vi "lib Variant to String.vi"(8 "error in (no error)":errorcluster, 11 "Variant":variant) -> (0 "error out":errorcluster, 3 "String":string)   [LabVIEW 2018]
uses:
  <vilib>/Utility/Data Type/NI_Data Type.lvlib
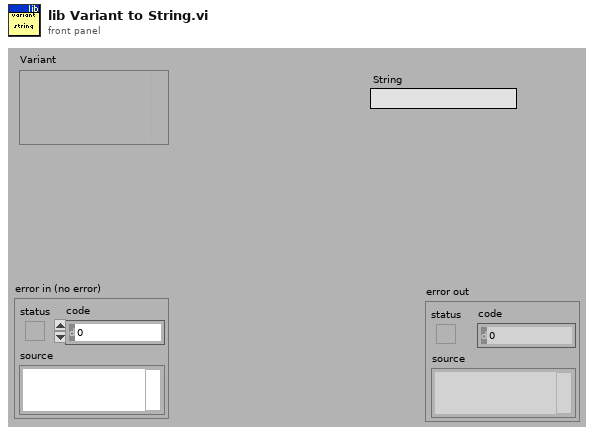
[diagram p1: front panel]
types:
  T1 = typedef "NI_Data Type.lvlib/Data Type.ctl" = enum8{"Invalid Type", "Void", "I8", "I16", "I32", "I64", "U8", "U16", "U32", "U64", "Single Float", "Double Float", "Extended Float", "Single Complex", "Double Complex", "Extended Complex", "Enum U8", "Enum U16", "Enum U32", "Enum U64", "Single Float With Unit", "Double Float With Unit", "Extended Float With Unit", "Single Complex with Unit", "Double Complex with Unit", "Extended Complex with Unit", "Boolean", "String", "Path", "Picture", "Tag", "Array", "Cluster", "Variant", "LV Variant", "Waveform", "Timestamp", "Digital Waveform", "Digital Data", "ExpressData", "Refnum", "External Data", "VI", "Poly VI", "LabVIEW Class Instance", "Fixed Point"}
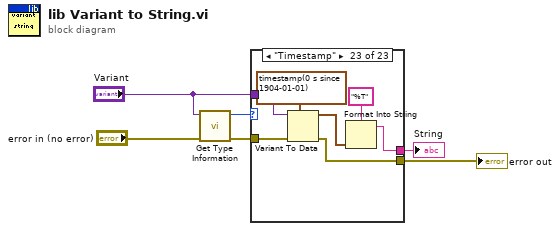
[diagram p0: block diagram]
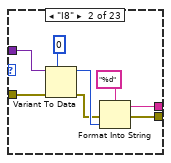
[diagram p3: hidden frame]
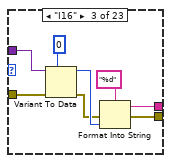
[diagram p4: hidden frame]
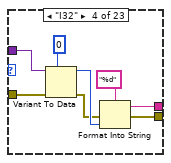
[diagram p5: hidden frame]
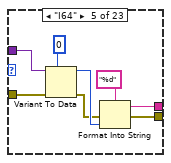
[diagram p6: hidden frame]
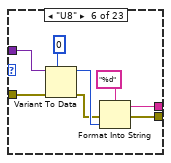
[diagram p7: hidden frame]
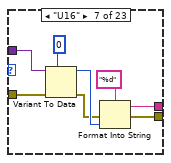
[diagram p8: hidden frame]
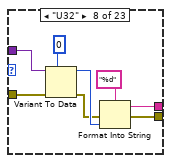
[diagram p9: hidden frame]
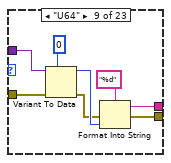
[diagram p10: hidden frame]
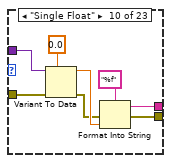
[diagram p11: hidden frame]
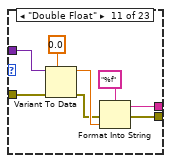
[diagram p12: hidden frame]
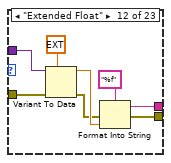
[diagram p13: hidden frame]
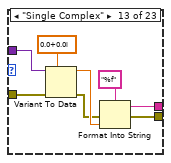
[diagram p14: hidden frame]
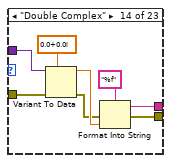
[diagram p15: hidden frame]
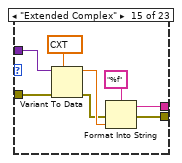
[diagram p16: hidden frame]
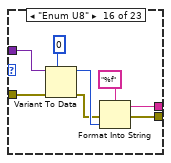
[diagram p17: hidden frame]
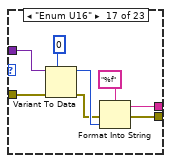
[diagram p18: hidden frame]
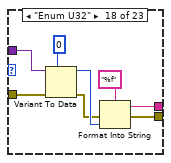
[diagram p19: hidden frame]
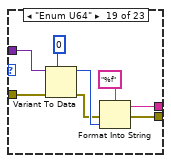
[diagram p20: hidden frame]
diagram:
  n1 = call <vilib>:"Get Type Information.vi"("error in (no error)"="error in (no error)", "Variant"="Variant") -> ("error out"=w5:errorcluster, "Type"=w6:T1)  [unwired: 5 in, 3 out]
  n2 = case shown="\"Timestamp\"" w6 {
    tunnel: "Variant" -> [_ w14 w22 w30 w38 w46 w54 w62 w70 w78 w86 w94 w102 w110 w118 w126 w134 w142 w150 w158 w163 w169 w176]
    tunnel: [_ w11 w19 w27 w35 w43 w51 w59 w67 w75 w83 w91 w99 w107 w115 w123 w131 w139 w147 w155 w160 w165 w171] -> w1
    tunnel: w5 -> [w7 w10 w18 w26 w34 w42 w50 w58 w66 w74 w82 w90 w98 w106 w114 w122 w130 w138 w146 w154 w162 w168 w175]
    tunnel: [w7 w8 w16 w24 w32 w40 w48 w56 w64 w72 w80 w88 w96 w104 w112 w120 w128 w136 w144 w152 w161 w166 w174] -> w2
    frame "Invalid Type", Default {
    }
    frame "I8" {
      n3 = Variant To Data(error in=w10, type=i8 0, Variant=w14) -> (data=w12:i8, error out=w9:errorcluster)
      n4 = Format Into String(format string="%d", error in=w9, w12) -> (resulting string=w11:string, error out=w8:errorcluster)  [unwired: 1 in]
    }
    frame "I16" {
      n5 = Variant To Data(error in=w18, type=i16 0, Variant=w22) -> (data=w20:i16, error out=w17:errorcluster)
      n6 = Format Into String(format string="%d", error in=w17, w20) -> (resulting string=w19:string, error out=w16:errorcluster)  [unwired: 1 in]
    }
    frame "I32" {
      n7 = Variant To Data(error in=w26, type=0, Variant=w30) -> (data=w28:i32, error out=w25:errorcluster)
      n8 = Format Into String(format string="%d", error in=w25, w28) -> (resulting string=w27:string, error out=w24:errorcluster)  [unwired: 1 in]
    }
    frame "I64" {
      n9 = Variant To Data(error in=w34, type=i64 0, Variant=w38) -> (data=w36:i64, error out=w33:errorcluster)
      n10 = Format Into String(format string="%d", error in=w33, w36) -> (resulting string=w35:string, error out=w32:errorcluster)  [unwired: 1 in]
    }
    frame "U8" {
      n11 = Variant To Data(error in=w42, type=u8 0, Variant=w46) -> (data=w44:u8, error out=w41:errorcluster)
      n12 = Format Into String(format string="%d", error in=w41, w44) -> (resulting string=w43:string, error out=w40:errorcluster)  [unwired: 1 in]
    }
    frame "U16" {
      n13 = Variant To Data(error in=w50, type=u16 0, Variant=w54) -> (data=w52:u16, error out=w49:errorcluster)
      n14 = Format Into String(format string="%d", error in=w49, w52) -> (resulting string=w51:string, error out=w48:errorcluster)  [unwired: 1 in]
    }
    frame "U32" {
      n15 = Variant To Data(error in=w58, type=u32 0, Variant=w62) -> (data=w60:u32, error out=w57:errorcluster)
      n16 = Format Into String(format string="%d", error in=w57, w60) -> (resulting string=w59:string, error out=w56:errorcluster)  [unwired: 1 in]
    }
    frame "U64" {
      n17 = Variant To Data(error in=w66, type=u64 0, Variant=w70) -> (data=w68:u64, error out=w65:errorcluster)
      n18 = Format Into String(format string="%d", error in=w65, w68) -> (resulting string=w67:string, error out=w64:errorcluster)  [unwired: 1 in]
    }
    frame "Single Float" {
      n19 = Variant To Data(error in=w74, type=sgl 0.0, Variant=w78) -> (data=w76:sgl, error out=w73:errorcluster)
      n20 = Format Into String(format string="%f", error in=w73, w76) -> (resulting string=w75:string, error out=w72:errorcluster)  [unwired: 1 in]
    }
    frame "Double Float" {
      n21 = Variant To Data(error in=w82, type=0.0, Variant=w86) -> (data=w84:dbl, error out=w81:errorcluster)
      n22 = Format Into String(format string="%f", error in=w81, w84) -> (resulting string=w83:string, error out=w80:errorcluster)  [unwired: 1 in]
    }
    frame "Extended Float" {
      n23 = Variant To Data(error in=w90, type=ext 0.0, Variant=w94) -> (data=w92:ext, error out=w89:errorcluster)
      n24 = Format Into String(format string="%f", error in=w89, w92) -> (resulting string=w91:string, error out=w88:errorcluster)  [unwired: 1 in]
    }
    frame "Single Complex" {
      n25 = Variant To Data(error in=w98, type=csg 0.0+0.0i, Variant=w102) -> (data=w100:csg, error out=w97:errorcluster)
      n26 = Format Into String(format string="%f", error in=w97, w100) -> (resulting string=w99:string, error out=w96:errorcluster)  [unwired: 1 in]
    }
    frame "Double Complex" {
      n27 = Variant To Data(error in=w106, type=cdb 0.0+0.0i, Variant=w110) -> (data=w108:cdb, error out=w105:errorcluster)
      n28 = Format Into String(format string="%f", error in=w105, w108) -> (resulting string=w107:string, error out=w104:errorcluster)  [unwired: 1 in]
    }
    frame "Extended Complex" {
      n29 = Variant To Data(error in=w114, type=cxt 0.0+0.0i, Variant=w118) -> (data=w116:cxt, error out=w113:errorcluster)
      n30 = Format Into String(format string="%f", error in=w113, w116) -> (resulting string=w115:string, error out=w112:errorcluster)  [unwired: 1 in]
    }
    frame "Enum U8" {
      n31 = Variant To Data(error in=w122, type=u8 0, Variant=w126) -> (data=w124:u8, error out=w121:errorcluster)
      n32 = Format Into String(format string="%f", error in=w121, w124) -> (resulting string=w123:string, error out=w120:errorcluster)  [unwired: 1 in]
    }
    frame "Enum U16" {
      n33 = Variant To Data(error in=w130, type=u16 0, Variant=w134) -> (data=w132:u16, error out=w129:errorcluster)
      n34 = Format Into String(format string="%f", error in=w129, w132) -> (resulting string=w131:string, error out=w128:errorcluster)  [unwired: 1 in]
    }
    frame "Enum U32" {
      n35 = Variant To Data(error in=w138, type=u32 0, Variant=w142) -> (data=w140:u32, error out=w137:errorcluster)
      n36 = Format Into String(format string="%f", error in=w137, w140) -> (resulting string=w139:string, error out=w136:errorcluster)  [unwired: 1 in]
    }
    frame "Enum U64" {
      n37 = Variant To Data(error in=w146, type=u64 0, Variant=w150) -> (data=w148:u64, error out=w145:errorcluster)
      n38 = Format Into String(format string="%f", error in=w145, w148) -> (resulting string=w147:string, error out=w144:errorcluster)  [unwired: 1 in]
    }
    frame "Boolean" {
      n39 = Variant To Data(error in=w154, type=TRUE, Variant=w158) -> (data=w156:bool, error out=w153:errorcluster)
      n40 = Format Into String(format string="%d", error in=w153, w156) -> (resulting string=w155:string, error out=w152:errorcluster)  [unwired: 1 in]
    }
    frame "String" {
      n41 = Variant To Data(error in=w162, type="", Variant=w163) -> (data=w160:string, error out=w161:errorcluster)
    }
    frame "Path" {
      n42 = Variant To Data(error in=w168, type=path "", Variant=w169) -> (data=w167:path, error out=w166:errorcluster)
      n43 = Path To String(path=w167) -> (string=w165:string)
    }
    frame "Timestamp" {
      n44 = Variant To Data(error in=w175, type=timestamp(0 s since 1904-01-01), Variant=w176) -> (data=w172:timestamp, error out=w174:errorcluster)
      n45 = Format Into String(format string="%T", w172) -> (resulting string=w171:string)  [unwired: 2 in, 1 out]
    }
  }
  "error out" <- w2
  "String" <- w1
